vi "Codec_CMD_0_Will.vi"(8 "error in (no error)":errorcluster, 10 "CMD":u32, 11 "SecureMqttCodec in":refnum<class "SecureMqttCodec.lvclass">) -> (0 "error out":errorcluster, 2 "<JSON>":string, 3 "SecureMqttCodec out":refnum<class "SecureMqttCodec.lvclass">)   [LabVIEW 2020, in "SecureMqttCodec.lvclass"]
uses:
  SecureMqttCodec.lvclass
  SecureMqttCodec.lvclass/SecureMqttCodec.ctl
  <vilib>/addons/JSON API/JSON Value/Set from JSON string.vi
  <vilib>/addons/JSON API/JSON Scalar/JSON Scalar.lvclass
  C:/Program Files/National Instruments/LabVIEW 2020/vi.lib/addons/JSON API/JSON Value/JSON Value.lvclass
  <vilib>/addons/JSON API/JSON Array/JSON Array.lvclass
  <vilib>/addons/JSON API/JSON Scalar/Set U32.vi
  <vilib>/addons/JSON API/JSON Scalar/Set String.vi
  <vilib>/addons/JSON API/JSON Array/Set JSON Array.vi
  <vilib>/addons/JSON API/JSON Value/Get as JSON string (pretty).vi
  <vilib>/addons/JSON API/JSON Value/JSON Value.lvclass
  <vilib>/addons/JSON API/Get Polymorphic/JSON GetSet.lvlib
panel:
  # "Command:\n0 -- Reg Client\n65535 -- Reg Will"
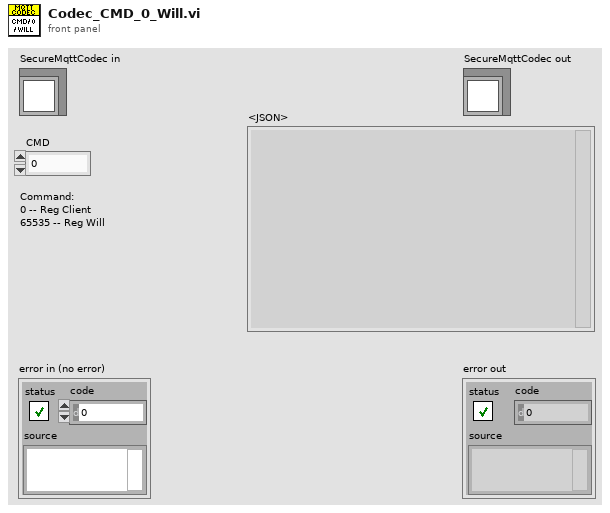
[diagram p1: front panel]
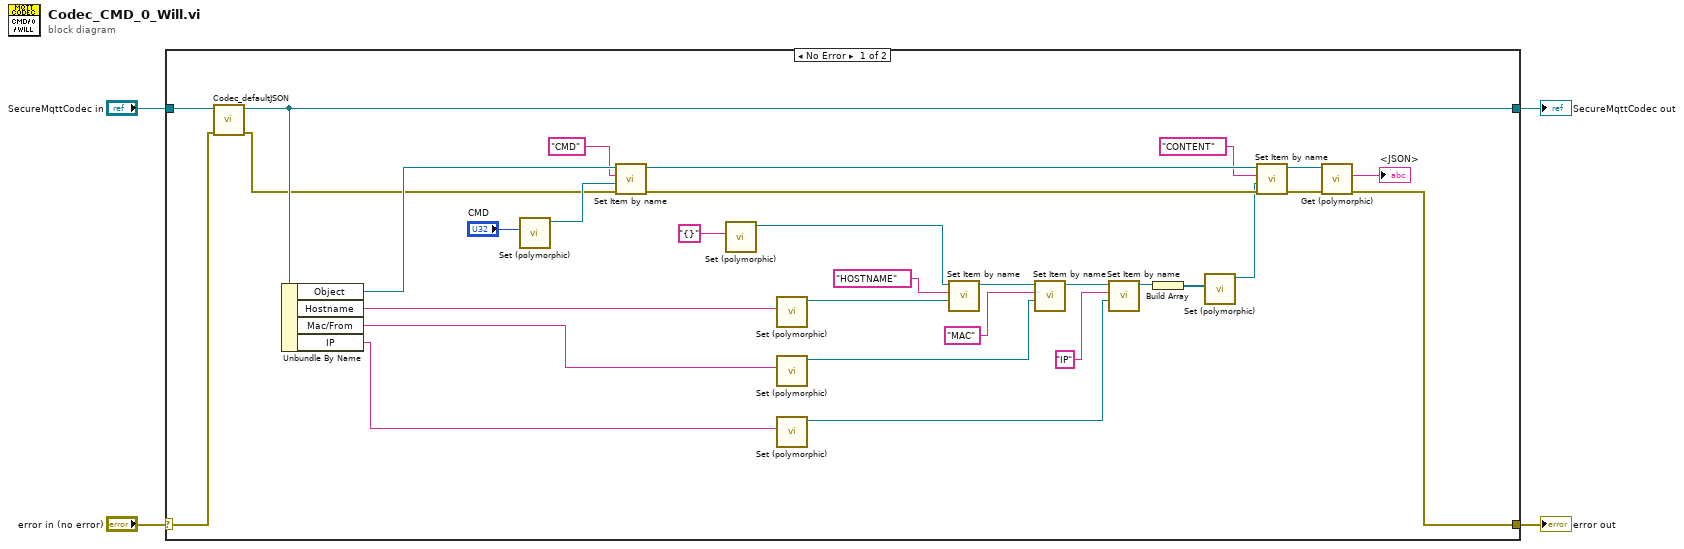
[diagram p0: block diagram]
diagram:
  n1 = case shown="No Error" "error in (no error)" {
    selector: "error in (no error)" -> [w5 w37]
    tunnel: [w30 w37] -> w3
    tunnel: [w7 w36] -> w1
    tunnel: "SecureMqttCodec in" -> [w35 w36]
    frame No Error {
      n2 = call "Codec_defaultJSON.vi"("error in (no error)"=w5, "SecureMqttCodec in"=w35) -> ("error out"=w6:errorcluster, "SecureMqttCodec out"=w7:refnum<class "SecureMqttCodec.lvclass">)  [unwired: 8 in]
      n3 = Unbundle By Name(w7) -> ("Object"=w34:refnum<class "JSON Value.lvclass">, "Hostname"=w16:string, "Mac/From"=w15:string, "IP"=w14:string)
      n4 = call-poly <vilib>:"Set (polymorphic).vi"("Numeric"="CMD") -> ("JSON Scalar out"=w32:refnum<class "JSON Scalar.lvclass">)  [unwired: 9 in, 1 out]
      n5 = call-dynamic "Set Item by name.vi"("error in (no error)"=w6, "Value"=w32, "name"="CMD", "JSON Value In"=w34) -> ("error out"=w11:errorcluster, "JSON Value Out"=w13:refnum<class "JSON Value.lvclass">)  [unwired: 5 in, 1 out]
      n6 = call-poly <vilib>:"Set (polymorphic).vi"("JSON stream"="{}" ("JSON")) -> ("JSON Value out"=w28:refnum<class "JSON Value.lvclass">)  [unwired: 8 in, 2 out]
      n7 = call-poly <vilib>:"Set (polymorphic).vi"("String"=w16) -> ("JSON Scalar out"=w27:refnum<class "JSON Scalar.lvclass">)  [unwired: 9 in, 1 out]
      n8 = call-poly <vilib>:"Set (polymorphic).vi"("String"=w15) -> ("JSON Scalar out"=w24:refnum<class "JSON Scalar.lvclass">)  [unwired: 9 in, 1 out]
      n9 = call-poly <vilib>:"Set (polymorphic).vi"("String"=w14) -> ("JSON Scalar out"=w23:refnum<class "JSON Scalar.lvclass">)  [unwired: 9 in, 1 out]
      n10 = call-dynamic "Set Item by name.vi"("Value"=w27, "name"="HOSTNAME", "JSON Value In"=w28) -> ("JSON Value Out"=w26:refnum<class "JSON Value.lvclass">)  [unwired: 6 in, 2 out]
      n11 = call-dynamic "Set Item by name.vi"("Value"=w24, "name"="MAC", "JSON Value In"=w26) -> ("JSON Value Out"=w25:refnum<class "JSON Value.lvclass">)  [unwired: 6 in, 2 out]
      n12 = call-dynamic "Set Item by name.vi"("Value"=w23, "name"="IP", "JSON Value In"=w25) -> ("JSON Value Out"=w22:refnum<class "JSON Value.lvclass">)  [unwired: 6 in, 2 out]
      n13 = Build Array(w22) -> (w21:refnum<class "JSON Value.lvclass">[])
      n14 = call-poly <vilib>:"Set (polymorphic).vi"("Array"=w21) -> ("JSON Array out"=w9:refnum<class "JSON Array.lvclass">)  [unwired: 9 in, 1 out]
      n15 = call-dynamic "Set Item by name.vi"("error in (no error)"=w11, "Value"=w9, "name"="CONTENT", "JSON Value In"=w13) -> ("error out"=w10:errorcluster, "JSON Value Out"=w12:refnum<class "JSON Value.lvclass">)  [unwired: 5 in, 1 out]
      n16 = call-poly <vilib>:"Get (polymorphic).vi"("error in (no error)"=w10, "JSON Value in"=w12) -> ("error out"=w30:errorcluster, "<JSON>"=→"<JSON>":string)  [unwired: 8 in]
    }
    frame Error {
    }
  }
  "error out" <- w3
  "SecureMqttCodec out" <- w1
